vi "get all batch statistcs.vi"(11 "ref in":T1) -> (3 "ref out":T1)   [LabVIEW 2024]
uses:
  CTRLS/REF.ctl
  CTRLS/Main Tabs.ctl
  CTRLS/Open Batch Data.ctl
  CTRLS/DM_Data.ctl
  CTRLS/run statistics.ctl
  CTRLS/System settings.ctl
  CTRLS/Printer Message settings.ctl
  CTRLS/Serial status Enum.ctl
  CTRLS/Serials DB Operations Enum.ctl
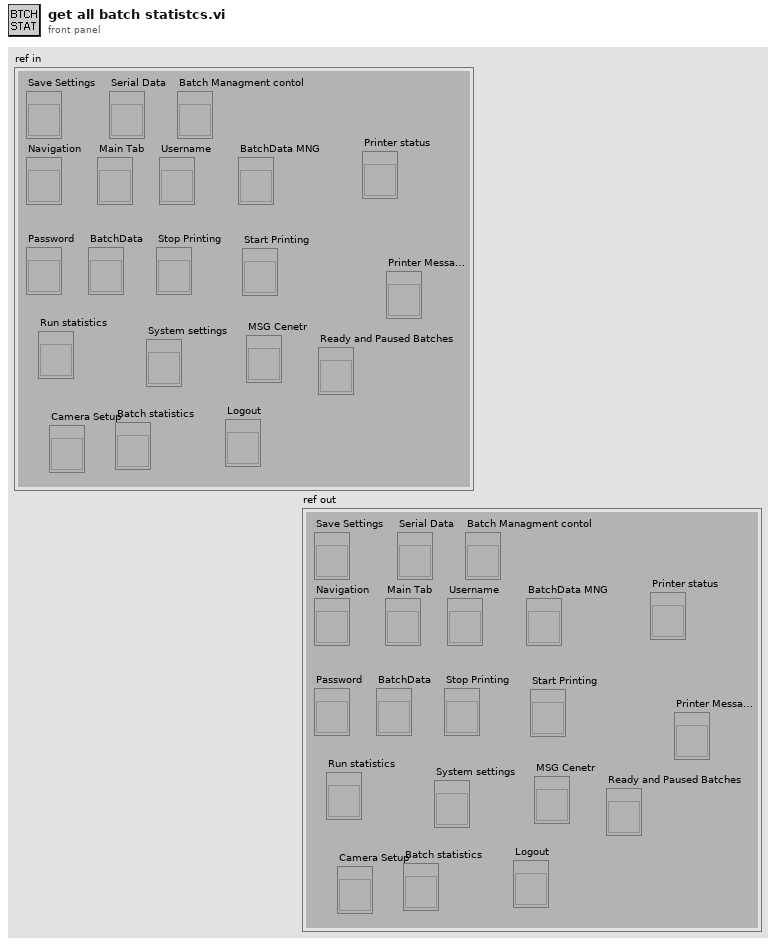
[diagram p1: front panel]
types:
  T1 = typedef "REF.ctl" = cluster{"Save Settings":refnum<vi>, "Navigation":refnum<vi>, "Main Tab":refnum<vi>, "Password":refnum<vi>, "BatchData":refnum<vi>, "Serial Data":refnum<vi>, "Username":refnum<vi>, "Stop Printing":refnum<vi>, "Run statistics":refnum<vi>, "System settings":refnum<vi>, "Batch Managment contol":refnum<vi>, "Start Printing":refnum<vi>, "BatchData MNG":refnum<vi>, "MSG Cenetr":refnum<vi>, "Printer status":refnum<vi>, "Printer Message Config":refnum<vi>, "Ready and Paused Batches":refnum<vi>, "Camera Setup":refnum<vi>, "Batch statistics":refnum<vi>, "Logout":refnum<vi>}
  T2 = typedef "Serial status Enum.ctl" = enum16{"NOT USED", "PRINTED", "ACCEPTED", "REJECTED"}
  T3 = typedef "Serials DB Operations Enum.ctl" = enum16{"Update serial verify status", "Get serials Based on Status", "Insert serials", "Update serial print status", "Get all Batch Serials", "Get Serial Status"}
  T4 = typedef "run statistics.ctl" = cluster{"Good":dbl, "Bad":dbl, "Good %":dbl, "Bad %":dbl}
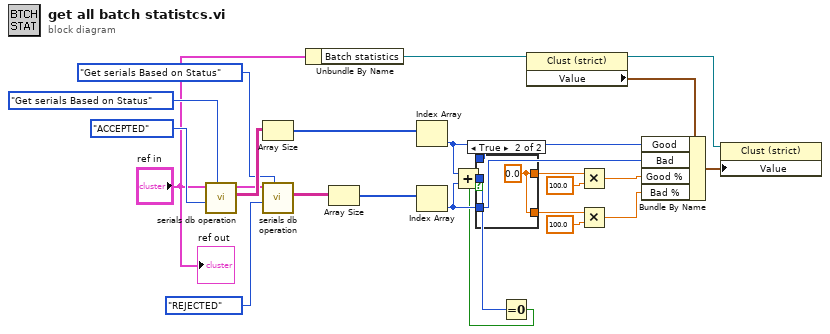
[diagram p0: block diagram]
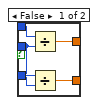
[diagram p2: hidden frame]
diagram:
  n1 = call "serials db operation.vi"("SRL DB OP"=Serials_DB_Operations_Enum."Get serials Based on Status", "Status"=Serial_status_Enum."ACCEPTED", "REF"="ref in") -> ("Fetched Serials"=w21:string[][], "REF out"=w15:T1)  [unwired: 5 in, 2 out]
  n2 = Array Size(array=w21) -> (size(s)=w20:i32[])
  n3 = call "serials db operation.vi"("SRL DB OP"=Serials_DB_Operations_Enum."Get serials Based on Status", "Status"=Serial_status_Enum."REJECTED", "REF"=w15) -> ("Fetched Serials"=w18:string[][])  [unwired: 5 in, 3 out]
  n4 = Unbundle By Name("ref in") -> ("Batch statistics"=w24:refnum<vi>)
  n5 = Array Size(array=w18) -> (size(s)=w19:i32[])
  n6 = Index Array(array=w20) -> (element=w11:i32)  [unwired: 1 in]
  n7 = Index Array(array=w19) -> (element=w5:i32)  [unwired: 1 in]
  n8 = Add(x=w11, y=w5) -> (x+y=w2:i32)
  n9 = Equal To 0?(x=w2) -> (x = 0?=w1:bool)
  n10 = case shown="True" w1 {
    tunnel: w11 -> [w29 _]
    tunnel: [w28 w30] -> w10
    tunnel: [w27 w30] -> w6
    tunnel: w5 -> [w26 _]
    tunnel: w2 -> [w25 _]
    frame False {
      n11 = Divide(x=w29, y=w25) -> (x/y=w28:dbl)
      n12 = Divide(x=w26, y=w25) -> (x/y=w27:dbl)
    }
    frame True {
      w30 = 0.0
    }
  }
  n13 = property class="Clust (strict)"(reference=w24) -> (reference out=w12:refnum<vi>, "Value"=w14:T4)  [unwired: 1 in, 1 out]
  n14 = Multiply(x=w10, y=100.0) -> (x*y=w8:dbl)
  n15 = Multiply(x=w6, y=100.0) -> (x*y=w4:dbl)
  n16 = Bundle By Name(cluster=w14, "Good"=w11, "Bad"=w5, "Good %"=w8, "Bad %"=w4) -> (w13:T4)
  n17 = property class="Clust (strict)"(reference=w12, "Value"=w13) -> ()  [unwired: 1 in, 2 out]
  "ref out" <- "ref in"
